vi "CIPT_softwarecontrol with trigger.vi"() -> ()   [LabVIEW 2022 SP3]
uses:
  Git/CIPT/CIPT/Labview Project/CIPT modes.ctl
  <vilib>/Analysis/baseanly.llb/Mean (DBL).vi
  <vilib>/Utility/file.llb/Read Delimited Spreadsheet (DBL).vi
  <vilib>/Utility/file.llb/Read Delimited Spreadsheet (I64).vi
  <vilib>/gmath/NumericalOptimization/Nonlinear Curve Fit LM.vi
  <vilib>/Utility/file.llb/Write Delimited Spreadsheet (string).vi
  <vilib>/Utility/file.llb/Write Delimited Spreadsheet (I64).vi
  <vilib>/Utility/file.llb/Write Delimited Spreadsheet (DBL).vi
  C:/CIPT/Labview Project/Camera Driver/Labview Driver/OtherDrivers/LabVIEW/ueye.NET/uEyeDotNet.dll
  CIPT/Labview Project/Camera Driver/Labview Driver/OtherDrivers/LabVIEW/ueye.NET/uEyeDotNet.dll
  <vilib>/gmath/NI_Gmath.lvlib
  <instrlib>/Keithley DMM6500 DAQ6500 Series/Keithley DMM6500 DAQ6500 Series.lvlib
  <instrlib>/Keithley 24XX/Keithley 24XX.lvlib
  <instrlib>/Keithley 2182/Keithley 2182.lvlib
  <vilib>/Analysis/NI_AALBase.lvlib
panel:
  out "Comms Errors":errorcluster[](array[cluster])
  in  "Save Filr":bool
  out "error file out":errorcluster
  in  "output file path":path=path "C:/CIPT/Labview Project/csv files/test output.csv"
  in  "stop":bool
  in  "Tab Control":T1(tab)
  in  "Camera ID 3":enum16{"2", "1"}(ring)
  in  "Camera ID 1":enum16{"2", "1"}(ring)
  in  "down a2":bool
  in  "up a2":bool
  in  "down a1":bool
  in  "up a1":bool
  in  "down a3":bool
  in  "up a3":bool
  in  "down all":bool
  in  "up all":bool
  in  "steps /\n continuous \ntoggle":bool
  out "Image first camera":picture
  out "Serial Number 1":string
  in  "Init Camera":bool
  in  "Exit Camera":bool
  in  "Init Camera 2":bool
  in  "Exit Camera 2":bool
  out "Serial Number 2":string
  out "Image second camera":picture
  out "Error Camera 1":errorcluster caption="error"
  out "Error Camera 2":errorcluster caption="error"
  in  "COM 1":refnum<visa-resource-name>
  out "error":errorcluster
  in  "Probe Landing File":path=path "C:/CIPT/Labview Project/csv files/Probe Landing cipt.csv"
  in  "Landing Test on/off?":bool
  in  "load file":bool
  in  "Step size":i32=10
  out "Resistance":dbl[][](array[numeric])
  out "Measurment":sgl[](array[numeric])
  out "Loaded":bool
  out "Loaded":bool
  out "Error Probe Configuration File":errorcluster
  in  "Probe Configuration File":path=path "C:/CIPT/Labview Project/csv files/test probe config.csv"
  in  "Probe Settings File":path=path "C:/CIPT/Labview Project/csv files/deafult_probe_setrings.CSV"
  out "Error Probe Settings File":errorcluster
  out "Probe Spacings":dbl[][](array[numeric])
  in  "Load":bool
  in  "Multiplexer":refnum<visa-resource-name>
  out "all rows":i64[][](array[numeric])
  out "Results Description":string[](array[string])
  out "Results":dbl[][](array[numeric])
  out "Probe Set 2":i32
  in  "Compliance voltage (V)":dbl=42.0
  in  "Measure Instrument":refnum<visa-resource-name>
  in  "Radio Buttons":T2 caption="Select Instrumentation"
  in  "Source Instrument":refnum<visa-resource-name>
  in  "Run":bool
  in  "Current (µA)":dbl=10.0
  out "Measurement Log":string
  out "Probe Set":i32
  in  "Measurement Repeats":i32=10
  in  "Size Of Buffer":i32=3
  in  "Time For Buffer To Fill(ms)":u32=2000
  in  "Top Film R est.":dbl=0.25
  in  "Bottm Film R est.":dbl=0.25
  in  "RA est.":dbl=0.25
  out "Top Film R":dbl
  out "Bottom Film R":dbl
  out "RA":dbl
  out "error out (fitting model)":errorcluster
  in  "Fit Data":bool
  out "Measurements Map Out":map{string, dbl[]}(c390)
  # "Probe Landing cipt_probe check: checks probes individually \nProbe Landing cipt: checks for any connection"
  # "All"
  # "End"
  # "home"
  # "Delete"
  # "Insert"
  # "Page Down"
  # "Page up"
  # "F2"
  # "F1"
  # "Steps"
  # "Continuous"
  # "Probe Settings"
  # "Probe Configuration"
  # "I+"
  # "V+"
  # "V-"
  # "I-"
  # "Max Resolution of 2400 is 300 µV in 200 mV range"
  # "/"
  # "Sheet Resistance (RA)"
  # "Estimated Values"
  # "Fitted Values"
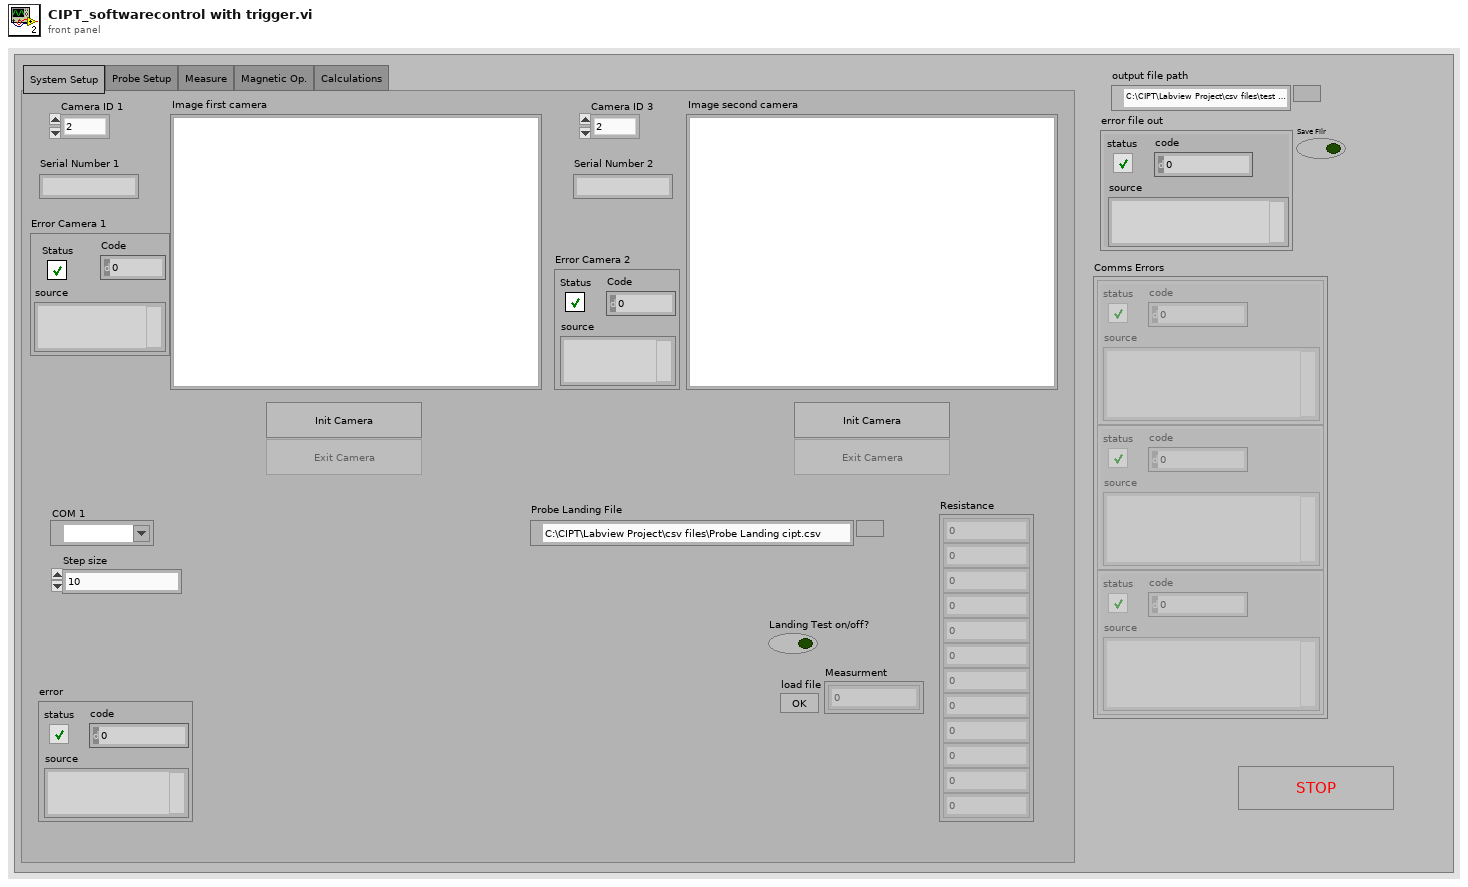
[diagram p1: front panel]
types:
  T1 = enum32{"System Setup", "Probe Setup", "Measure", "Magnetic Op.", "Calculations"}
  T2 = typedef "CIPT modes.ctl" = enum32{"DAQ6510", "2400 Only", "2400 and  2182", "SR830", "SR830 and 6221"}
  T3 = enum32{"System Setup", "Probe Setup", "Measure", "Magnetic Operations", "Calculations + Analyis"}
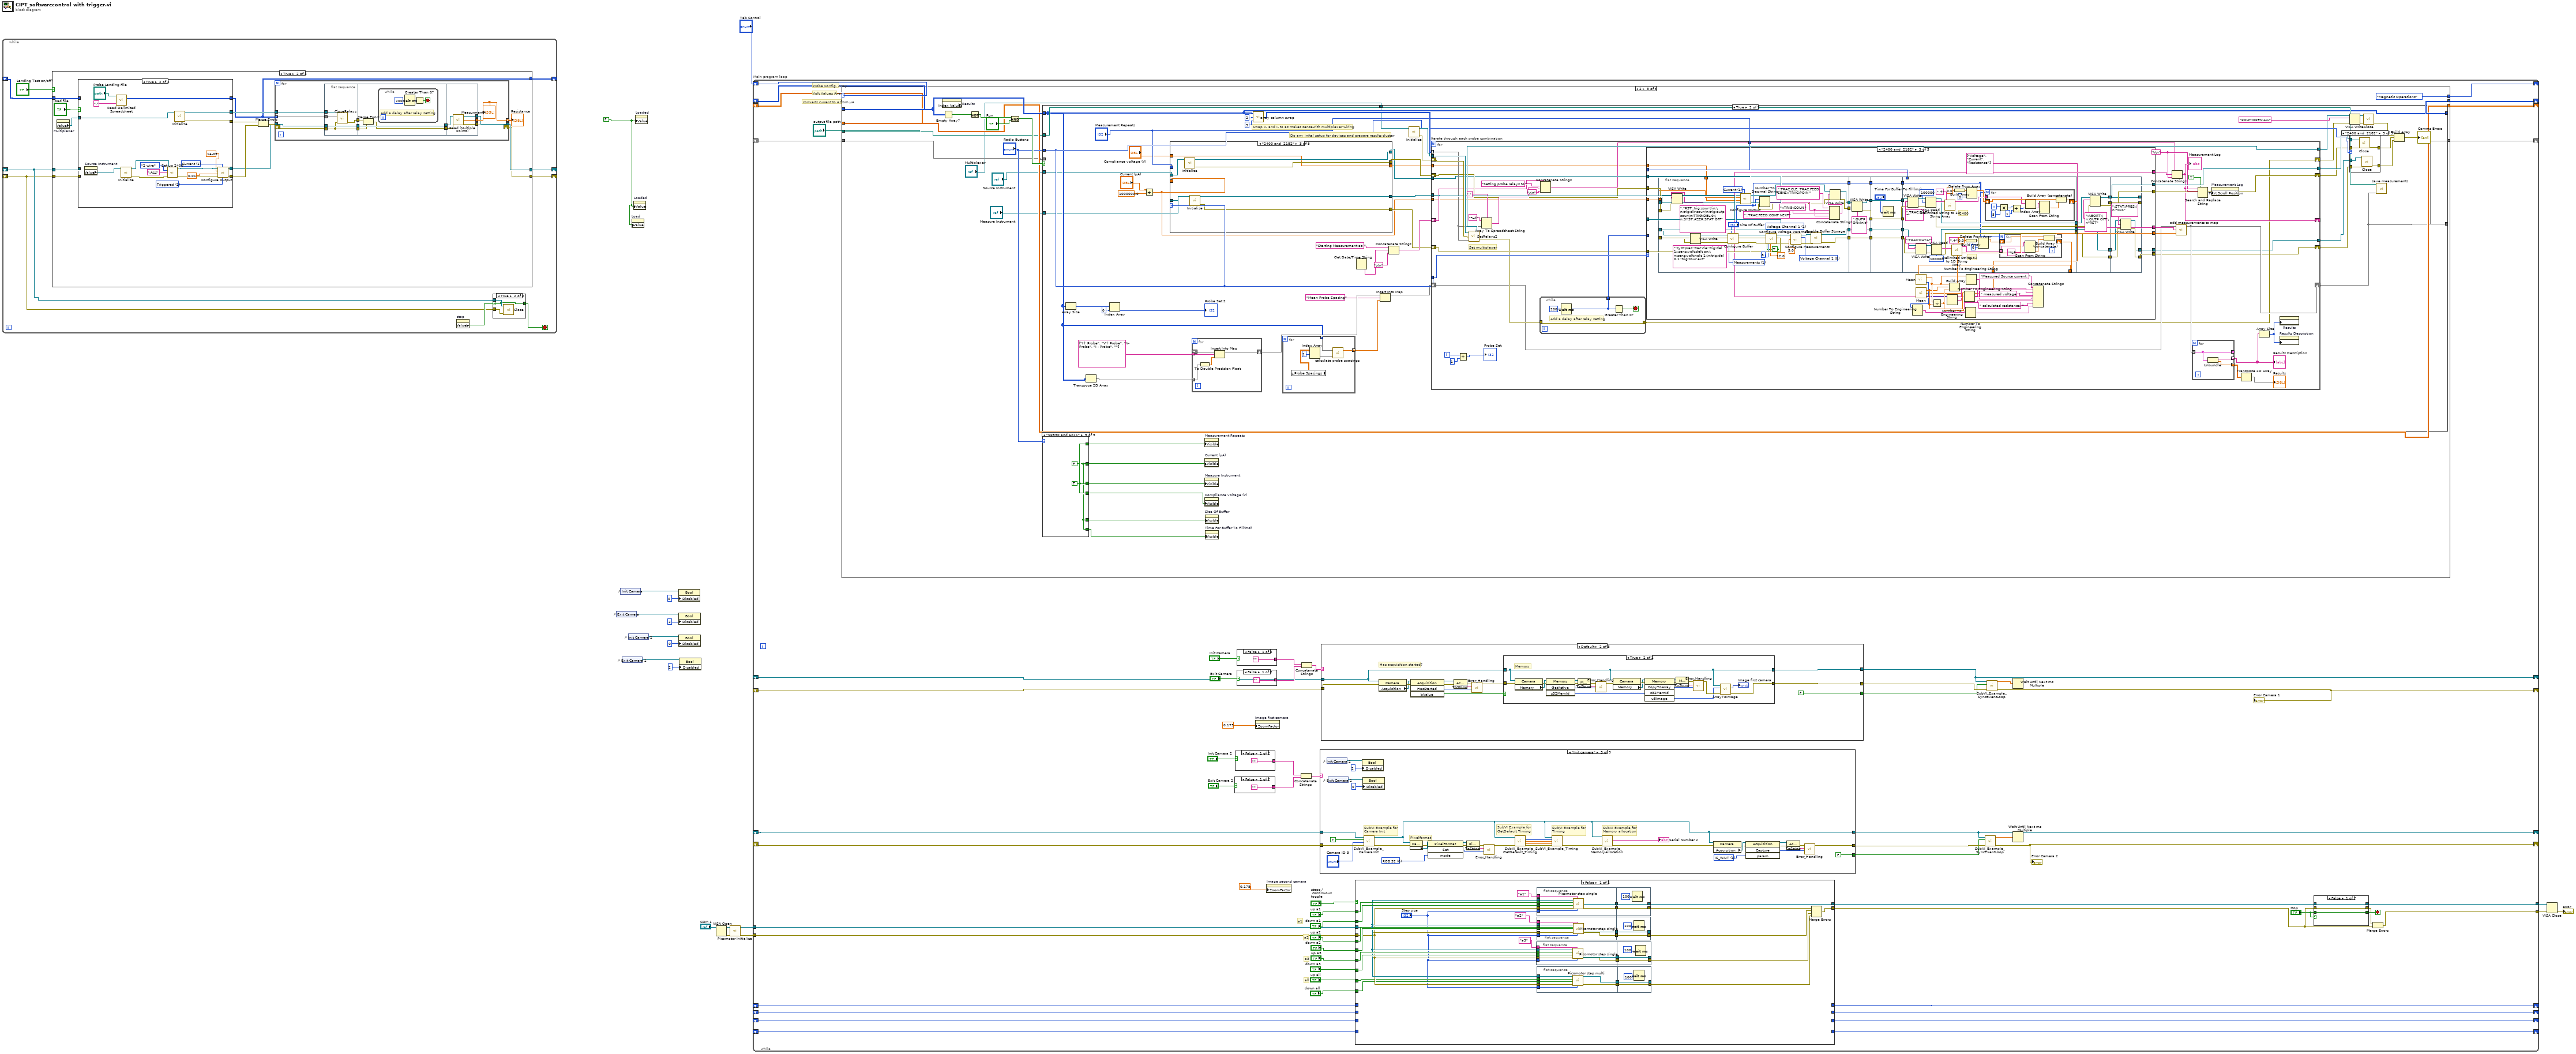
[diagram p0: block diagram]
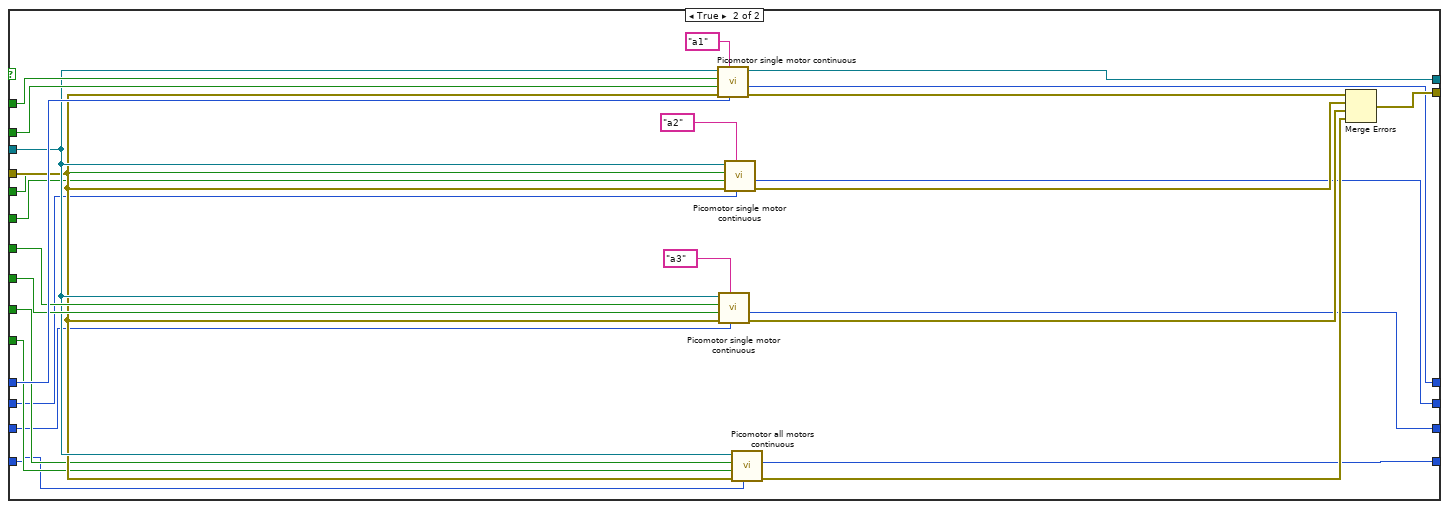
[diagram p5: hidden frame]
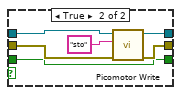
[diagram p6: hidden frame]
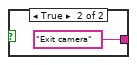
[diagram p7: hidden frame]
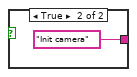
[diagram p8: hidden frame]
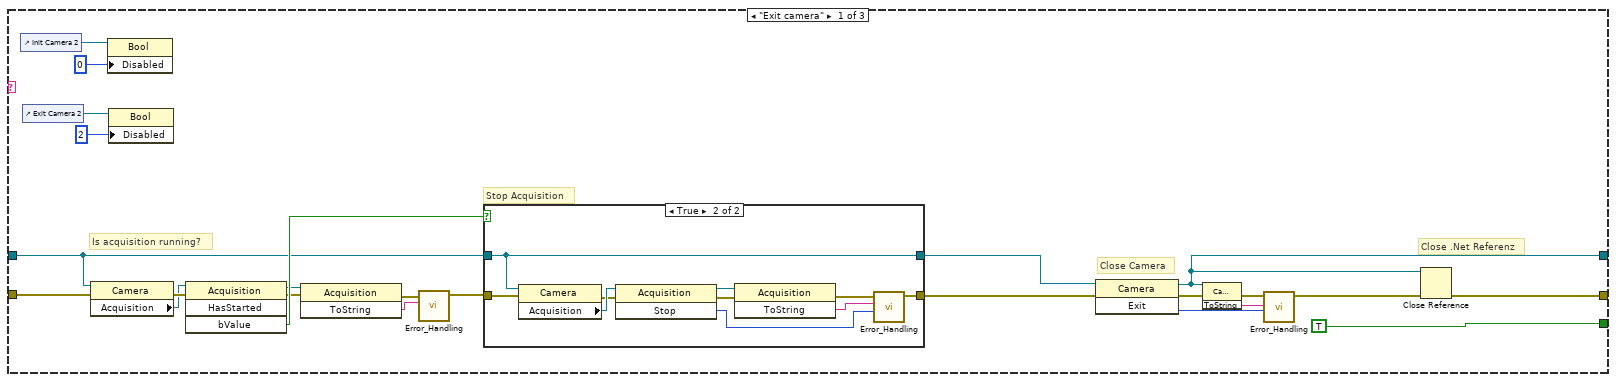
[diagram p9: hidden frame]
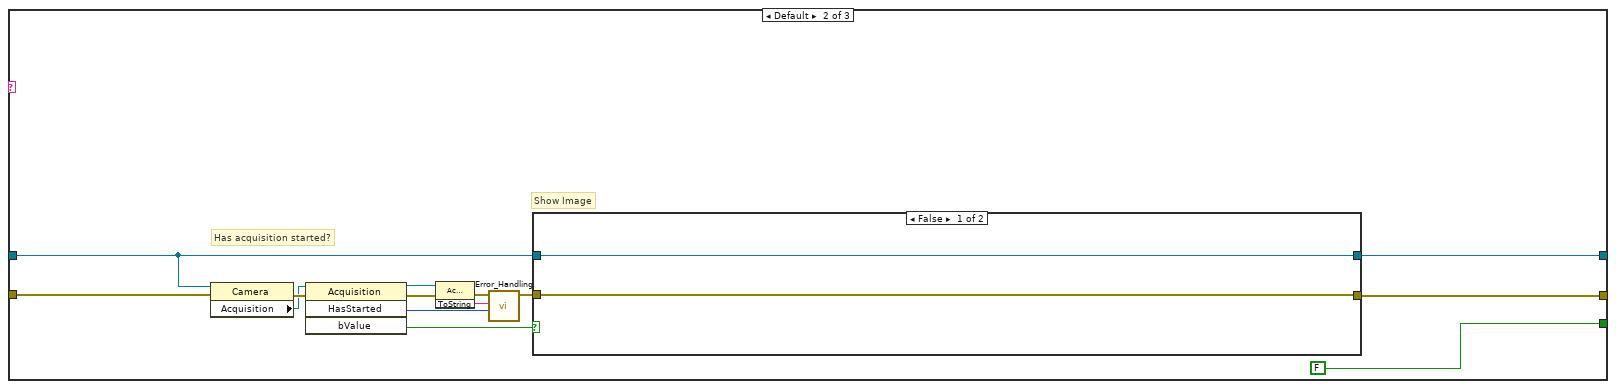
[diagram p11: hidden frame]
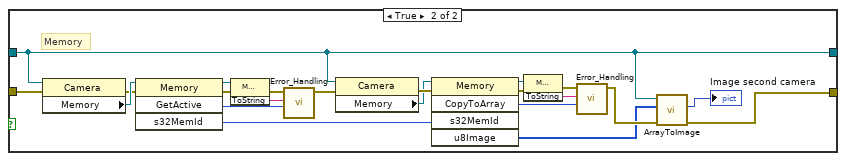
[diagram p12: hidden frame]
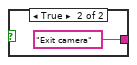
[diagram p13: hidden frame]
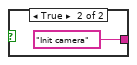
[diagram p14: hidden frame]
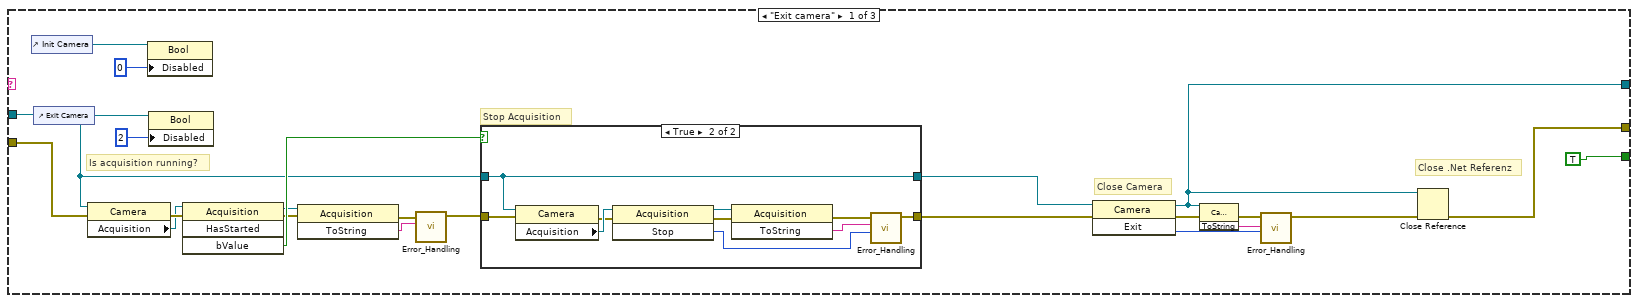
[diagram p15: hidden frame]
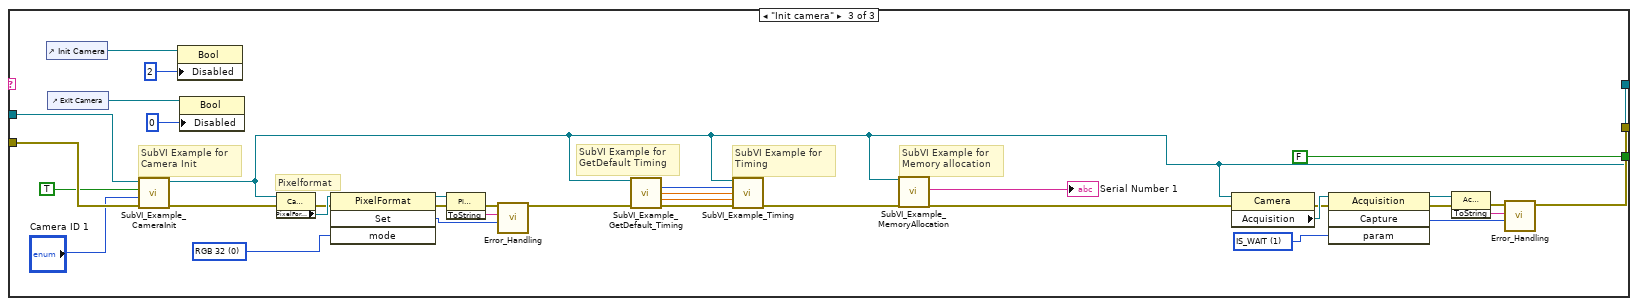
[diagram p18: hidden frame]
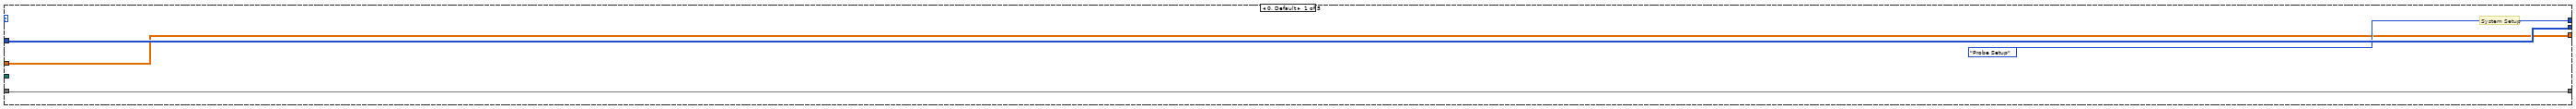
[diagram p19: hidden frame]
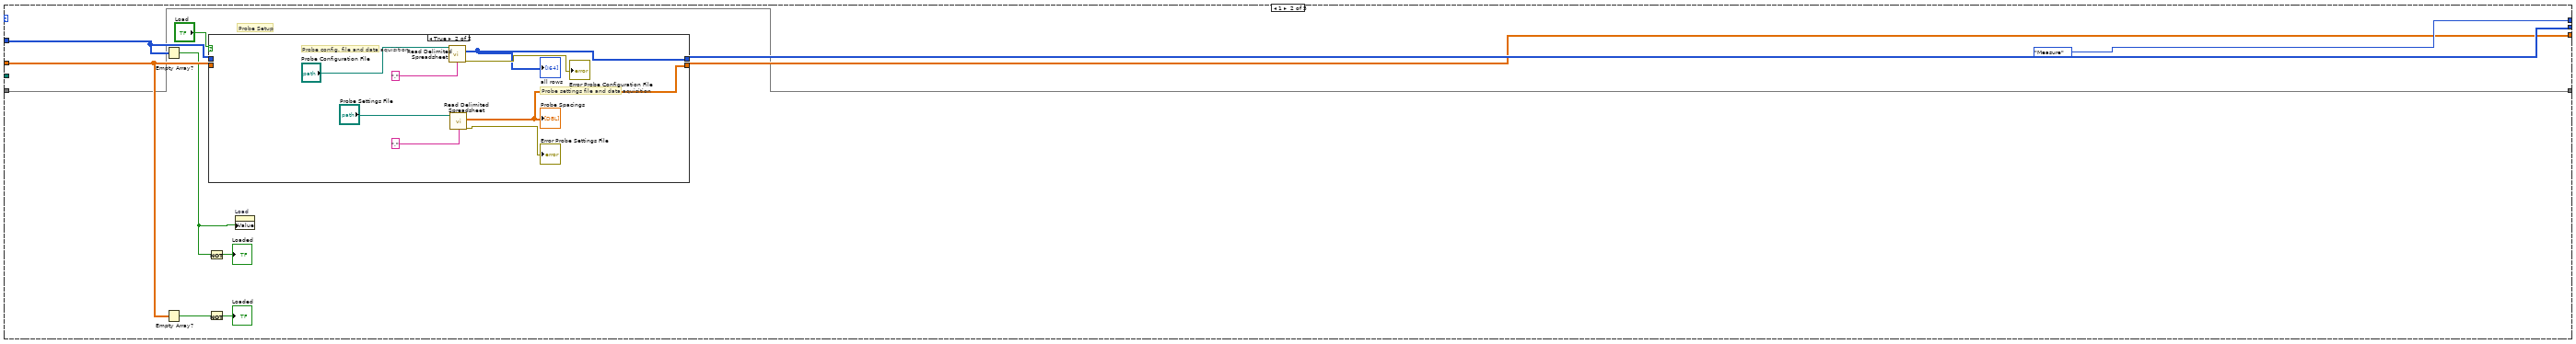
[diagram p20: hidden frame]
diagram:
  w9 = FALSE
  n1 = while {
    shift-right: [w26] -> _
    shift-left: _ -> [w23]
    shift-right: [w25] -> _
    shift-left: _ -> [w22]
    shift-right: [w20] -> _
    shift-left: _ -> [w19]
    stop <- w21 stop-if-true
    n2 = case shown="True" "Landing Test on/off?" {
      tunnel: w23 -> [w34 w43]
      tunnel: w22 -> [w33 w42]
      tunnel: [w34 w41] -> w26
      tunnel: [w33 w40] -> w25
      tunnel: w19 -> [w32 w36]
      tunnel: [w32 w35] -> w20
      frame False {
      }
      frame True {
        n3 = property on="Multiplexer" class="VISAName"() -> ("Value"=w39:refnum<visa-resource-name>)  [unwired: 2 in, 2 out]
        n4 = case shown="True" "load file" {
          tunnel: [_ w84] -> w48
          tunnel: [w80 w87] -> w45
          tunnel: [w81 w86] -> w44
          tunnel: w43 -> [w81 _]
          tunnel: w42 -> [w80 _]
          tunnel: [w79 w85] -> w38
          tunnel: w39 -> [w79 w83]
          tunnel: [w78 w82] -> w35
          tunnel: w36 -> [w78 _]
          frame False {
          }
          frame True {
            w93 = u16 1 items=["Immediate", "Triggered"] ("Output Type  (0: Immediate)")
            w92 = u16 1 items=["Voltage", "Current"] ("Source Mode  (0: Voltage)")
            n5 = property on="Source Instrument" class="VISAName"() -> ("Value"=w98:refnum<visa-resource-name>)  [unwired: 2 in, 2 out]
            n6 = call-poly <vilib>:"Read Delimited Spreadsheet.vi"("file path (dialog if empty)"="Probe Landing File", "delimiter (\\t)"="," ("delimiter (\\t)")) -> ("all rows"=w82:i64[][])  [unwired: 8 in, 5 out]
            n7 = call <instrlib>:"Initialize.vi"("VISA resource name"=w98) -> ("error out"=w95:errorcluster, "VISA resource name out"=w94:refnum<visa-resource-name>)  [unwired: 9 in]
            n8 = call "Set up 2400.vi"("VISA resource name"=w94, "Sense mode"=enum16{"2 wire", "4 wire"}."2 wire", "Measurement Function"=":ALL", "error in (no error)"=w95) -> ("VISA resource name out"=w96:refnum<visa-resource-name>, "error out"=w97:errorcluster)  [unwired: 10 in]
            n9 = call <instrlib>:"Initialize.vi"("VISA resource name"=w83) -> ("error out"=w84:errorcluster, "VISA resource name out"=w85:refnum<visa-resource-name>)  [unwired: 9 in]
            n10 = call <instrlib>:"Configure Output.vi"("Output Type  (0: Immediate)"=w93, "Source Mode  (0: Voltage)"=w92, "error in (no error)"=w97, "Compliance  Level (0.1)"=0.01, "Output Level (0)"=1e-05, "VISA resource name"=w96) -> ("error out"=w87:errorcluster, "VISA resource name out"=w86:refnum<visa-resource-name>)  [unwired: 4 in]
          }
        }
        n11 = Merge Errors(w48, w45) -> (w47:errorcluster)
        n12 = for {
          tunnel: [w54] -> w37 mode=indexing
          tunnel: w38 -> [w50]
          shift-right: [w51] -> w40
          shift-left: w47 -> [w55]
          tunnel: w35 -> [w49] mode=indexing
          tunnel: w44 -> [w53]
          tunnel: [w52] -> w41
          n13 = flat-sequence {
            tunnel: w53 -> [w65]
            tunnel: w55 -> [w61]
            tunnel: [w61] -> w60
            tunnel: [w65] -> w59
            tunnel: w50 -> [w64]
            tunnel: [w63] -> w58
            tunnel: w49 -> [w62]
            tunnel: [w67] -> w57
            tunnel: [w69] -> w56
            tunnel: w60 -> [w68]
            tunnel: w59 -> [w69]
            tunnel: w58 -> [w66]
            tunnel: [w75] -> w54
            tunnel: [w74] -> w52
            tunnel: [w73] -> w51
            tunnel: w57 -> [w77]
            tunnel: w56 -> [w76]
            frame #0 {
              n14 = call "CloseRelays.vi"("error in (no error)"=w61, "Array"=w62, "VISA Refnum in"=w64) -> ("error out"=w63:errorcluster)  [unwired: 6 in, 2 out]
            }
            frame #1 {
              n15 = Merge Errors(w66, w68) -> (w67:errorcluster)
              n16 = while {
                stop <- w71 stop-if-true
                # "Add a delay after relay setting"
                n17 = Wait (ms)(milliseconds to wait=u32 200) -> (millisecond timer value=w70:u32)
                n18 = Greater Than 0?(x=w70) -> (x > 0?=w71:bool)
              }
            }
            frame #2 {
              n19 = call <instrlib>:"Read (Multiple Points).vi"("VISA resource name"=w76, "error in (no error)"=w77) -> ("VISA resource name out"=w74:refnum<visa-resource-name>, "Resistance"=w75:sgl[], "error out"=w73:errorcluster)  [unwired: 7 in, 4 out]
            }
          }
          "Measurment" <- w54
        }
        "Resistance" <- w37
      }
    }
    n20 = property on="stop" class="Bool (strict)"() -> ("Value"=w24:bool)  [unwired: 2 in, 2 out]
    n21 = case shown="True" w24 {
      selector: w24 -> [w28 w29]
      tunnel: w23 -> [_ w31]
      tunnel: w22 -> [_ w30]
      tunnel: [w28 w29] -> w21
      frame False {
      }
      frame True {
        n22 = call <instrlib>:"Close.vi"("error in (no error)"=w30, "VISA resource name"=w31) -> ()  [unwired: 9 in, 1 out]
      }
    }
  }
  n23 = control-ref of="Exit Camera"() -> (w12:refnum<vi>)
  n24 = control-ref of="Init Camera"() -> (w13:refnum<vi>)
  n25 = control-ref of="Exit Camera 2"() -> (w17:refnum<vi>)
  n26 = control-ref of="Init Camera 2"() -> (w16:refnum<vi>)
  n27 = property on="Load" class="Bool (strict)"("Value"=w9) -> ()  [unwired: 2 in, 2 out]
  n28 = property on="Loaded" class="Bool (strict)"("Value"=w9) -> ()  [unwired: 2 in, 2 out]
  n29 = property on="Loaded" class="Bool (strict)"("Value"=w9) -> ()  [unwired: 2 in, 2 out]
  n30 = property class="Bool"(reference=w13, "Disabled"=u8 0 ("Deaktiviert")) -> ()  [unwired: 1 in, 2 out]
  n31 = property class="Bool"(reference=w12, "Disabled"=u8 2 ("Deaktiviert")) -> ()  [unwired: 1 in, 2 out]
  n32 = property class="Bool"(reference=w16, "Disabled"=u8 0 ("Deaktiviert")) -> ()  [unwired: 1 in, 2 out]
  n33 = property class="Bool"(reference=w17, "Disabled"=u8 2 ("Deaktiviert")) -> ()  [unwired: 1 in, 2 out]
  n34 = VISA Open(VISA resource name="COM 1") -> (VISA resource name=w7:refnum<visa-resource-name>, error out=w6:errorcluster)  [unwired: 4 in]
  n35 = call "Picomotor Initialize.vi"("error in (no error)"=w6, "VISA Refnum in"=w7) -> ("error out"=w4:errorcluster, "VISA Refnum out"=w5:refnum<visa-resource-name>)  [unwired: 8 in]
  n36 = while "Main program loop" {
    shift-right: [w159] -> _
    shift-left: _ -> [w160]
    shift-right: [w158] -> _
    shift-left: "Tab Control" -> [w161]
    shift-right: [w157] -> _
    shift-left: _ -> [w156]
    shift-right: [w154] -> _
    shift-left: _ -> [w153]
    shift-right: [w142] -> _
    shift-left: _ -> [w140]
    shift-right: [w143] -> _
    shift-left: _ -> [w141]
    shift-right: [w130] -> _
    shift-left: _ -> [w128]
    shift-right: [w129] -> _
    shift-left: _ -> [w127]
    tunnel: w5 -> [w114]
    tunnel: w4 -> [w113]
    tunnel: [w126] -> w2
    shift-right: [w111] -> _
    shift-left: _ -> [w107]
    shift-right: [w110] -> _
    shift-left: _ -> [w106]
    shift-right: [w109] -> _
    shift-left: _ -> [w105]
    shift-right: [w108] -> _
    shift-left: _ -> [w104]
    tunnel: [w101] -> w1
    stop <- w125 stop-if-true
    # "a2"
    # "a3"
    # "all"
    # "a1"
    # "converts current to A from µA"
    # "Volt Values Array"
    # "Probe Config. Array"
    n37 = case shown="2" w161 {
      tunnel: w160 -> [w500 w507 w538 w895 w902]
      tunnel: [w500 w511 w537 w895 w902] -> w159
      tunnel: [T3."Probe Setup" ("Tab Control") T3."Measure" ("Tab Control") T3."Magnetic Operations" ("Tab Control") T3."Calculations + Analyis" ("Tab Control") T3."System Setup" ("Tab Control")] -> w158
      tunnel: [w498 w506 w532 w894 w901] -> w157
      tunnel: w156 -> [w498 w505 w532 w894 w901]
      tunnel: "output file path" -> [_ _ w530 _ w900]
      tunnel: [w497 w502 w529 w893 w899] -> w154
      tunnel: w153 -> [w497 w502 w528 w893 w899]
      frame 0, Default {
        # "System Setup"
      }
      frame 1 {
        # "Probe Setup"
        n38 = Empty Array?(array=w507) -> (empty?=w501:bool)
        n39 = Empty Array?(array=w505) -> (empty?=w504:bool)
        n40 = Not(x=w501) -> (.not. x?=→"Loaded":bool)
        n41 = Not(x=w504) -> (.not. x?=→"Loaded":bool)
        n42 = case shown="True" "Load" {
          tunnel: [w513 w514] -> w511
          tunnel: w507 -> [w513 _]
          tunnel: [w512 w515] -> w506
          tunnel: w505 -> [w512 _]
          frame False {
          }
          frame True {
            # "Probe config. file and data aquisition"
            # "Probe settings file and data aquisition"
            n43 = call-poly <vilib>:"Read Delimited Spreadsheet.vi"("file path (dialog if empty)"="Probe Configuration File", "delimiter (\\t)"="," ("delimiter (\\t)")) -> ("all rows"=w514:i64[][], "error out"=→"Error Probe Configuration File":errorcluster)  [unwired: 8 in, 4 out]
            "all rows" <- w514
            n44 = call-poly <vilib>:"Read Delimited Spreadsheet.vi"("file path (dialog if empty)"="Probe Settings File", "delimiter (\\t)"="," ("delimiter (\\t)")) -> ("all rows"=w515:dbl[][], "error out"=→"Error Probe Settings File":errorcluster)  [unwired: 8 in, 4 out]
            "Probe Spacings" <- w515
          }
        }
        n45 = property on="Load" class="Bool (strict)"("Value"=w501) -> ()  [unwired: 2 in, 2 out]
      }
      frame 2 {
        n46 = property on="Results" class="Arr (strict)" props=["Index Values"]() -> ()  [unwired: 2 in, 3 out]
        n47 = Empty Array?(array=w538) -> (empty?=w540:bool)
        n48 = Not(x=w540) -> (.not. x?=w539:bool)
        n49 = Compound Arithmetic op=AND(w539, "Run") -> (w542:bool)
        n50 = case shown="True" w542 {
          tunnel: w538 -> [w553 w572]
          tunnel: [w553 w572] -> w537
          tunnel: "Radio Buttons" -> [_ w598]
          tunnel: w530 -> [_ w586]
          tunnel: [w552 w568] -> w529
          tunnel: w528 -> [w552 _]
          tunnel: "Measure Instrument" -> [_ w560]
          tunnel: "Source Instrument" -> [_ w559]
          tunnel: "Multiplexer" -> [_ w558]
          frame False {
          }
          frame True {
            # "Swap V- and I- to as makes sensewith multiplexer wiring"
            # "Do any inital setup for devices and prepare results cluster"
            n51 = Array Size(array=w572) -> (size(s)=w592:i32[])
            n52 = Transpose 2D Array(2D array=w572) -> (transposed array=w571:i64[][])
            n53 = Index Array "Index Array"(array=w592, index=0) -> (element=→"Probe Set 2":i32)
            n54 = Divide(x="Current (µA)", y=1000000.0) -> (x/y=w554:dbl)
            n55 = case shown="\"2400 and  2182\"" w598 {
              tunnel: w559 -> [_ w636 w642 _ _]
              tunnel: [_ w624 w641 _ _] -> w599
              tunnel: w560 -> [_ _ w643 _ _]
              tunnel: [_ w624 w639 _ _] -> w562
              tunnel: [_ w630 w638 _ _] -> w593
              tunnel: w554 -> [_ w627 _ _ _]
              tunnel: "Compliance voltage (V)" -> [_ w625 w637 _ _]
              tunnel: "Measurement Repeats" -> [_ _ _ _ _]
              tunnel: [_ _ w640 _ _] -> w557
              tunnel: [_ _ w637 _ _] -> w555
              frame "DAQ6510", Default {
              }
              frame "2400 Only" {
                w628 = u16 1 items=["Immediate", "Triggered"] ("Output Type  (0: Immediate)")
                w629 = u16 1 items=["Voltage", "Current"] ("Source Mode  (0: Voltage)")
                n56 = call <instrlib>:"Initialize.vi"("VISA resource name"=w636) -> ("error out"=w634:errorcluster, "VISA resource name out"=w635:refnum<visa-resource-name>)  [unwired: 9 in]
                n57 = call "Set up 2400.vi"("VISA resource name"=w635, "Sense mode"=enum16{"2 wire", "4 wire"}."4 wire", "Measurement Function"=":ALL", "error in (no error)"=w634) -> ("VISA resource name out"=w632:refnum<visa-resource-name>, "error out"=w631:errorcluster)  [unwired: 10 in]
                n58 = call <instrlib>:"Configure Output.vi"("Output Type  (0: Immediate)"=w628, "Source Mode  (0: Voltage)"=w629, "error in (no error)"=w631, "Compliance  Level (0.1)"=w625, "Output Level (0)"=w627, "VISA resource name"=w632) -> ("error out"=w630:errorcluster, "VISA resource name out"=w624:refnum<visa-resource-name>)  [unwired: 4 in]
              }
              frame "2400 and  2182" {
                n59 = call <instrlib>:"Initialize.vi"("VISA resource name"=w642) -> ("error out"=w638:errorcluster, "VISA resource name out"=w639:refnum<visa-resource-name>)  [unwired: 9 in]
                n60 = call <instrlib>:"Initialize.vi"("VISA resource name"=w643) -> ("error out"=w640:errorcluster, "VISA resource name out"=w641:refnum<visa-resource-name>)  [unwired: 9 in]
              }
              frame "SR830" {
              }
              frame "SR830 and 6221" {
              }
            }
            n61 = for {
              tunnel: w571 -> [w610] mode=indexing
              tunnel: string[] ["I+ Probe", "V+ Probe", "V- Probe", "I - Probe", ""] -> [w611] mode=indexing
              shift-right: [w608] -> w576
              shift-left: _ -> [w607]
              n62 = To Double Precision Float(number=w610) -> (double precision float=w609:dbl[])
              n63 = Insert Into Map(map in=w607, key=w611, value=w609) -> (map out=w608:map{string, dbl[]})  [unwired: 2 out]
            }
            n64 = call "array column swap.vi"("Collumn 2 index"=3, "Collumn 1 index"=2, "Input array"=w572) -> ("output array"=w589:i32[][])
            n65 = for {
              tunnel: w572 -> [w603] mode=indexing
              tunnel: [w602] -> w575 mode=indexing
              n66 = local read "Probe Spacings"() -> (w606:dbl[][])
              n67 = Index Array(array=w606, index (row)=1) -> (element=w604:dbl[])  [unwired: 1 in]
              n68 = call "calculate probe spacings.vi"("Probe Spacings"=w604, "Probe list"=w603) -> ("Mean Spacing"=w602:dbl)  [unwired: 1 out]
            }
            n69 = Get Date/Time String() -> (time string=w595:string)  [unwired: 3 in, 1 out]
            n70 = Insert Into Map(map in=w576, key="Mean Probe Spacing", value=w575) -> (map out=w573:map{string, dbl[]})  [unwired: 2 out]
            n71 = Concatenate Strings("Starting Measurement at: ", w595, "\r\n") -> (w584:string)
            n72 = call <instrlib>:"Initialize.vi"("VISA resource name"=w558) -> ("error out"=w600:errorcluster, "VISA resource name out"=w601:refnum<visa-resource-name>)  [unwired: 9 in]
            n73 = for "Iterate through each probe combination" {
              tunnel: w601 -> [w685]
              tunnel: [w684] -> w582
              tunnel: w589 -> [w678] mode=indexing
              tunnel: w598 -> [w683]
              tunnel: w599 -> [w681]
              shift-right: [w667] -> _
              shift-left: w584 -> [w668]
              shift-right: [w679] -> w596
              shift-left: w593 -> [w672]
              shift-right: [w658] -> w568
              shift-left: w573 -> [w660]
              shift-right: [w651] -> w569
              shift-left: w557 -> [w652]
              tunnel: w562 -> [w671]
              tunnel: [w680] -> w597
              shift-right: [w654] -> w564
              shift-left: w600 -> [w682]
              tunnel: [w650] -> w570
              tunnel: "Measurement Repeats" -> [w649]
              tunnel: w555 -> [w645]
              tunnel: w554 -> [w644]
              i -> [w648]
              w665 = "\r\n"
              # "Set multiplexer"
              n74 = Add(x=w648, y=1) -> (x+y=→"Probe Set":i32)
              n75 = call "SetRelays2.vi"("all rows"=w678, "error in (no error)"=w682, "VISA Refnum in"=w685) -> ("error out"=w673:errorcluster, "VISA resource name out"=w684:refnum<visa-resource-name>)  [unwired: 1 in]
              n76 = Array To Spreadsheet String(delimiter (Tab)=",", array=w678, 3:"%d" ("format string")) -> (spreadsheet string=w674:string)
              n77 = while {
                tunnel: [w692] -> w654
                tunnel: w673 -> [w692]
                tunnel: [w689] -> w653
                stop <- w690 stop-if-true
                # "Add a delay after relay setting"
                n78 = Wait (ms)(milliseconds to wait=u32 200) -> (millisecond timer value=w689:u32)
                n79 = Greater Than 0?(x=w689) -> (x > 0?=w690:bool)
              }
              n80 = Concatenate Strings(w668, "Setting probe relays to:", w674, "\r\n") -> (w663:string)
              n81 = case shown="\"2400 and  2182\"" w683 {
                tunnel: w681 -> [w694 w698 w763 w885 w889]
                tunnel: w671 -> [w693 w719 w771 w886 w890]
                tunnel: w672 -> [w695 w718 w770 w887 w891]
                tunnel: [w693 w716 w731 w886 w890] -> w680
                tunnel: [w695 w715 w739 w887 w891] -> w679
                tunnel: [_ w708 w764 _ _] -> w669
                tunnel: w649 -> [_ w707 w769 _ _]
                tunnel: [_ w701 w768 _ _] -> w661
                tunnel: [_ string[] ["Voltage", "Current", "Resistance"] string[] ["Voltage", "Current", "Resistance"] _ _] -> w662
                tunnel: w653 -> [_ _ _ _ _]
                tunnel: w652 -> [w696 w699 w762 w888 w892]
                tunnel: [w696 w699 w735 w888 w892] -> w651
                tunnel: [w694 w698 w732 w885 w889] -> w650
                tunnel: w645 -> [_ _ w724 _ _]
                tunnel: w644 -> [_ _ w723 _ _]
                frame "DAQ6510", Default {
                }
                frame "2400 Only" {
                  w717 = u16 0 items=["Fixed", "Sweep", "List"] ("Output Mode (0: Fixed)")
                  n82 = call <instrlib>:"Read (Multiple Points).vi"("VISA resource name"=w719, "Sample Count (1)"=w707, "error in (no error)"=w718, "Output Mode (0: Fixed)"=w717) -> ("Voltage"=w697:sgl[], "VISA resource name out"=w716:refnum<visa-resource-name>, "Current"=w706:sgl[], "Resistance"=w705:sgl[], "error out"=w715:errorcluster)  [unwired: 5 in, 2 out]
                  n83 = call-poly <vilib>:"Mean.vi"("X"=w697) -> ("mean"=w704:dbl)  [unwired: 1 out]
                  n84 = call-poly <vilib>:"Mean.vi"("X"=w706) -> ("mean"=w703:dbl)  [unwired: 1 out]
                  n85 = call-poly <vilib>:"Mean.vi"("X"=w705) -> ("mean"=w702:dbl)  [unwired: 1 out]
                  n86 = Build Array(w704, w703, w702) -> (w701:dbl[])
                  n87 = Number To Engineering String(4:w704) -> (0:w709:string)  [unwired: 3 in]
                  n88 = Number To Engineering String(4:w703) -> (0:w713:string)  [unwired: 3 in]
                  n89 = Number To Engineering String(4:w702) -> (0:w710:string)  [unwired: 3 in]
                  n90 = Concatenate Strings("Measured I = ", w713, " V = " ("string"), w709, "R = " ("string"), w710) -> (w708:string)
                }
                frame "2400 and  2182" {
                  n91 = flat-sequence {
                    tunnel: w762 -> [w785]
                    tunnel: w763 -> [w786]
                    tunnel: w770 -> [w778]
                    tunnel: w771 -> [w779]
                    tunnel: [w783] -> w734
                    tunnel: [w782] -> w733
                    tunnel: [w781] -> w726
                    tunnel: [w780] -> w725
                    tunnel: w724 -> [w776]
                    tunnel: w723 -> [w775]
                    tunnel: ["Size Of Buffer"] -> w720
                    tunnel: [w816] -> w751
                    tunnel: [w815] -> w749
                    tunnel: [w813] -> w746
                    tunnel: [w812] -> w744
                    tunnel: w734 -> [w816]
                    tunnel: w733 -> [w815]
                    tunnel: w726 -> [w814]
                    tunnel: w725 -> [_]
                    tunnel: [w810] -> w721
                    tunnel: w720 -> [w810]
                    tunnel: w751 -> [w822]
                    tunnel: [w822] -> w750
                    tunnel: w749 -> [w821]
                    tunnel: [w821] -> w748
                    tunnel: [w820] -> w747
                    tunnel: w746 -> [w820]
                    tunnel: [w819] -> w745
                    tunnel: w744 -> [w819]
                    tunnel: [w818] -> w722
                    tunnel: w721 -> [w818]
                    tunnel: w769 -> [_]
                    tunnel: w750 -> [w832]
                    tunnel: w748 -> [w831]
                    tunnel: w747 -> [w834]
                    tunnel: w745 -> [w833]
                    tunnel: [w830] -> w743
                    tunnel: [w829] -> w742
                    tunnel: [w827] -> w741
                    tunnel: [w826] -> w740
                    tunnel: [w825] -> w737
                    tunnel: [w824] -> w736
                    tunnel: w722 -> [w823]
                    tunnel: w741 -> [w877]
                    tunnel: w740 -> [w876]
                    tunnel: w737 -> [w872]
                    tunnel: w736 -> [w873]
                    tunnel: [w874] -> w730
                    tunnel: [w873] -> w729
                    tunnel: [w872] -> w728
                    tunnel: [w871] -> w727
                    tunnel: [w883] -> w731
                    tunnel: [w878] -> w732
                    tunnel: [w879] -> w735
                    tunnel: [w884] -> w739
                    tunnel: w730 -> [w884]
                    tunnel: w729 -> [w880]
                    tunnel: w728 -> [w881]
                    tunnel: w727 -> [w883]
                    frame #0 {
                      w787 = 0 items=["Voltage Channel 1", "Voltage Channel 2", "Temperature Channel 1", "Temperature Channel 2"] ("Measurement (0: Voltage Channel 1)")
                      w777 = u16 1 items=["Voltage", "Current"] ("Source Mode  (0: Voltage)")
                      w800 = 1 items=["Voltage Channel 1"=1, "Voltage Channel 2"=2] ("Measurement (1: Voltage Channel 1)")
                      w801 = 1 items=["None", "Measurements", "Math Calculation"] ("Buffer Source (0: None)")
                      n92 = VISA Write(VISA resource name=w779, write buffer=":*RST;:trig:sour tlin;\n:trig:dir sour;\n:trig:outp sour;\n:TRIG:DEL 0;\n:SYST:AZER:STAT OFF", error in (no error)=w778) -> (VISA resource name out=w796:refnum<visa-resource-name>, error out=w791:errorcluster)  [unwired: 1 out]
                      n93 = VISA Write(VISA resource name=w786, write buffer=":syst:pres;:trac:cle;:trig:del 1;:sens:volt:delt on;\n:sens:volt:nplc 1;\n:trig:del 0.1;:trig:sour ext", error in (no error)=w785) -> (VISA resource name out=w798:refnum<visa-resource-name>, error out=w797:errorcluster)  [unwired: 1 out]
                      n94 = call <instrlib>:"Configure Buffer.vi"("error in (no error)"=w797, "Buffer Source (0: None)"=w801, "Buffer Size (2)"="Size Of Buffer", "VISA resource name"=w798) -> ("error out"=w802:errorcluster, "VISA resource name out"=w805:refnum<visa-resource-name>)  [unwired: 6 in]
                      n95 = call <instrlib>:"Configure Output.vi"("Source Mode  (0: Voltage)"=w777, "error in (no error)"=w791, "Compliance  Level (0.1)"=w776, "Output Level (0)"=w775, "VISA resource name"=w796) -> ("error out"=w790:errorcluster, "VISA resource name out"=w774:refnum<visa-resource-name>)  [unwired: 5 in]
                      n96 = Number To Decimal String(number="Size Of Buffer") -> (decimal integer string=w792:string)  [unwired: 1 in]
                      n97 = call <instrlib>:"Configure Voltage Parameters.vi"("VISA resource name"=w805, "Measurement (1: Voltage Channel 1)"=w800, "Voltage Resolution (8)"=8, "Range Value (12)"=12.0, "Autorange (T: Enable)"=TRUE, "error in (no error)"=w802) -> ("VISA resource name out"=w804:refnum<visa-resource-name>, "error out"=w803:errorcluster)  [unwired: 8 in]
                      n98 = call <instrlib>:"Configure Measurements.vi"("VISA resource name"=w804, "Measurement (0: Voltage Channel 1)"=w787, "Integration Rate (5)"=5.0, "error in (no error)"=w803) -> ("VISA resource name out"=w789:refnum<visa-resource-name>, "error out"=w788:errorcluster)  [unwired: 10 in]
                      n99 = call <instrlib>:"Enable Buffer Storage.vi"("error in (no error)"=w788, "VISA resource name"=w789) -> ("error out"=w782:errorcluster, "VISA resource name out"=w783:refnum<visa-resource-name>)  [unwired: 8 in]
                      n100 = Concatenate Strings(":TRAC:CLE;:TRAC:FEED SENS;:TRAC:POIN " ("write buffer"), w792, ";:TRIG:COUN " ("write buffer"), w792, ";:TRAC:FEED:CONT NEXT" ("write buffer")) -> (w773:string)
                      n101 = VISA Write(VISA resource name=w774, write buffer=w773, error in (no error)=w790) -> (VISA resource name out=w781:refnum<visa-resource-name>, error out=w780:errorcluster)  [unwired: 1 out]
                    }
                    frame #1 {
                      n102 = VISA Write(VISA resource name=w814, write buffer=":OUTP ON;:init") -> (VISA resource name out=w813:refnum<visa-resource-name>, error out=w812:errorcluster)  [unwired: 1 in, 1 out]
                    }
                    frame #2 {
                      n103 = Wait (ms)(milliseconds to wait="Time For Buffer To Fill(ms)") -> ()  [unwired: 1 out]
                    }
                    frame #3 {
                      # "2182"
                      # "2400"
                      n104 = VISA Write(VISA resource name=w834, write buffer=":TRAC:DATA?", error in (no error)=w833) -> (VISA resource name out=w844:refnum<visa-resource-name>, error out=w843:errorcluster)  [unwired: 1 out]
                      n105 = VISA Write(VISA resource name=w832, write buffer=":TRAC:DATA?", error in (no error)=w831) -> (VISA resource name out=w853:refnum<visa-resource-name>, error out=w852:errorcluster)  [unwired: 1 out]
                      n106 = VISA Read(VISA resource name=w844, byte count=u32 100000, error in (no error)=w843) -> (VISA resource name out=w827:refnum<visa-resource-name>, read buffer=w840:string, error out=w826:errorcluster)  [unwired: 1 out]
                      n107 = VISA Read(VISA resource name=w853, byte count=u32 100000, error in (no error)=w852) -> (VISA resource name out=w825:refnum<visa-resource-name>, read buffer=w850:string, error out=w824:errorcluster)  [unwired: 1 out]
                      n108 = call <vilib>:"Delimited String to 1D String Array.vi"("delimiter"=",+" ("delimiter (Tab)"), "delimited string"=w840) -> ("string array"=w836:string[])  [unwired: 9 in]
                      n109 = call <vilib>:"Delimited String to 1D String Array.vi"("delimiter"=",+" ("delimiter (Tab)"), "delimited string"=w850) -> ("string array"=w845:string[])  [unwired: 9 in]
                      n110 = Build Array(0.0 ("array")) -> (w838:dbl[])
                      n111 = Build Array(0.0 ("array")) -> (w848:dbl[])
                      n112 = Delete From Array(array=w838, index=0) -> (array with subset deleted=w828:dbl[])  [unwired: 1 in, 1 out]
                      n113 = Delete From Array(array=w848, index=0) -> (array with subset deleted=w846:dbl[])  [unwired: 1 in, 1 out]
                      n114 = for {
                        N: w823 -> [_]
                        shift-right: [w859] -> w829
                        shift-left: w828 -> [w858]
                        tunnel: w836 -> [w857]
                        i -> [w865]
                        n115 = Multiply(x=w865, y=5) -> (x*y=w864:i32)
                        n116 = Add(x=w864, y=1) -> (x+y=w861:i32)
                        n117 = Index Array(array=w857, index=w861) -> (element=w856:string)
                        n118 = Scan From String(input string=w856) -> (output 1=w860:dbl)  [unwired: 4 in, 3 out]
                        n119 = Build Array (concatenate)(w858, w860) -> (w859:dbl[])
                      }
                      n120 = for {
                        N: w823 -> [_]
                        shift-right: [w868] -> w830
                        shift-left: w846 -> [w867]
                        tunnel: w845 -> [w866] mode=indexing
                        n121 = Scan From String(format string="%f", input string=w866) -> (output 1=w869:dbl)  [unwired: 3 in, 3 out]
                        n122 = Build Array (concatenate)(w867, w869) -> (w868:dbl[])
                      }
                    }
                    frame #4 {
                      n123 = VISA Write(VISA resource name=w877, write buffer=":ABORT;\n:OUTP OFF;\n*RST" ("data"), error in (no error)=w876) -> (VISA resource name out=w871:refnum<visa-resource-name>, error out=w874:errorcluster)  [unwired: 1 out]
                    }
                    frame #5 {
                      n124 = VISA Write(VISA resource name=w881, write buffer=":STAT:PRES;\n:*CLS" ("data"), error in (no error)=w880) -> (VISA resource name out=w878:refnum<visa-resource-name>, error out=w879:errorcluster)  [unwired: 1 out]
                    }
                  }
                  n125 = call-poly <vilib>:"Mean.vi"("X"=w743) -> ("mean"=w767:dbl, "error"=w755:i32)
                  n126 = Number To Engineering String(4:w755) -> (0:w754:string)  [unwired: 3 in]
                  n127 = call-poly <vilib>:"Mean.vi"("X"=w742) -> ("mean"=w766:dbl, "error"=w759:i32)
                  n128 = Divide(x=w767, y=w766) -> (x/y=w765:dbl)
                  n129 = Number To Engineering String(4:w759) -> (0:w758:string)  [unwired: 3 in]
                  n130 = Build Array(w767, w766, w765) -> (w768:dbl[])
                  n131 = Number To Engineering String(4:w766) -> (0:w760:string)  [unwired: 3 in]
                  n132 = Number To Engineering String(4:w765) -> (0:w752:string)  [unwired: 3 in]
                  n133 = Number To Engineering String(4:w767) -> (0:w756:string)  [unwired: 3 in]
                  n134 = Concatenate Strings("Measured Source current: " ("string"), w760, w758, " measured voltage: " ("string"), w756, w754, " calculated resistance: " ("string"), w752) -> (w764:string)
                }
                frame "SR830" {
                }
                frame "SR830 and 6221" {
                }
              }
              n135 = Concatenate Strings(w663, w669, w665) -> (w667:string)
              "Measurement Log" <- w667
              n136 = call "add measurements to map.vi"("Measurement Values"=w661, "Measurement Names"=w662, "Measurements Map in"=w660) -> ("Measurements Map Out"=w658:map{string, dbl[]})  [unwired: 2 in]
              n137 = for {
                tunnel: [w688] -> _ mode=indexing
                tunnel: w658 -> [w688] mode=indexing
                tunnel: [w687] -> w657 mode=indexing
                tunnel: [w686] -> w656 mode=indexing
                n138 = Unbundle(w688) -> (w687:string, "Array"=w686:dbl[])
              }
              "Results Description" <- w657
              n139 = Search and Replace String(replace all?=TRUE, input string=w667, search string=w665) -> (number of replacements=w664:i32)  [unwired: 5 in, 3 out]
              n140 = property on="Measurement Log" class="Str"("Text.Scroll Position"=w664) -> ()  [unwired: 2 in, 2 out]
              n141 = Transpose 2D Array(2D array=w656) -> (transposed array=→"Results":dbl[][])
              n142 = Array Size(array=w657) -> (size(s)=w659:i32)
              n143 = property on="Results" class="Arr (strict)"("Number of Columns"=w659) -> ()  [unwired: 2 in, 2 out]
              n144 = property on="Results Description" class="Arr (strict)"("Number of Columns"=w659) -> ()  [unwired: 2 in, 2 out]
            }
            n145 = VISA Write(VISA resource name=w582, write buffer="ROUT:OPEN:ALL", error in (no error)=w564) -> (VISA resource name out=w581:refnum<visa-resource-name>, error out=w580:errorcluster)  [unwired: 1 out]
            n146 = case shown="\"2400 and  2182\"" w598 {
              tunnel: w597 -> [_ w617 w622 _ _]
              tunnel: w596 -> [w613 w616 w623 _ _]
              tunnel: [w613 w615 w618 _ _] -> w567
              tunnel: w570 -> [_ _ w621 _ _]
              tunnel: w569 -> [w612 w614 w620 _ _]
              tunnel: [w612 w614 w619 _ _] -> w566
              frame "DAQ6510", Default {
              }
              frame "2400 Only" {
                n147 = call <instrlib>:"Close.vi"("error in (no error)"=w616, "VISA resource name"=w617) -> ("error out"=w615:errorcluster)  [unwired: 9 in]
              }
              frame "2400 and  2182" {
                n148 = call <instrlib>:"Close.vi"("error in (no error)"=w623, "VISA resource name"=w622) -> ("error out"=w618:errorcluster)  [unwired: 9 in]
                n149 = call <instrlib>:"Close.vi"("error in (no error)"=w620, "VISA resource name"=w621) -> ("error out"=w619:errorcluster)  [unwired: 9 in]
              }
              frame "SR830" {
              }
              frame "SR830 and 6221" {
              }
            }
            n150 = call <instrlib>:"Close.vi"("error in (no error)"=w580, "VISA resource name"=w581) -> ("error out"=w563:errorcluster)  [unwired: 9 in]
            n151 = call "save measurements.vi"("Save path"=w586, "Measurements In"=w568) -> ()  [unwired: 12 in, 2 out]
            n152 = Build Array(w563, w567, w566) -> (→"Comms Errors":errorcluster[])
          }
        }
        n153 = case shown="\"SR830 and 6221\"" "Radio Buttons" {
          tunnel: [w543 w545 w547 w548 w551] -> w536
          tunnel: [w543 w546 w547 w548 w550] -> w535
          tunnel: [TRUE w546 w547 TRUE w551] -> w531
          tunnel: [w543 w546 w547 w548 w551] -> w524
          tunnel: [w543 w545 w547 w548 w550] -> w523
          tunnel: [w543 w545 w547 w548 w550] -> w522
          frame "DAQ6510", Default {
            w543 = FALSE
          }
          frame "2400 Only" {
            w546 = TRUE
            w545 = FALSE
          }
          frame "2400 and  2182" {
            w547 = TRUE
          }
          frame "SR830" {
            w548 = FALSE
          }
          frame "SR830 and 6221" {
            w550 = FALSE
            w551 = TRUE
          }
        }
        n154 = property on="Measurement Repeats" class="DigNum (strict)"("Visible"=w531) -> ()  [unwired: 2 in, 2 out]
        n155 = property on="Current (µA)" class="DigNum (strict)"("Visible"=w535) -> ()  [unwired: 2 in, 2 out]
        n156 = property on="Measure Instrument" class="VISAName"("Visible"=w536) -> ()  [unwired: 2 in, 2 out]
        n157 = property on="Compliance voltage (V)" class="DigNum (strict)"("Visible"=w524) -> ()  [unwired: 2 in, 2 out]
        n158 = property on="Size Of Buffer" class="DigNum (strict)"("Visible"=w523) -> ()  [unwired: 2 in, 2 out]
        n159 = property on="Time For Buffer To Fill(ms)" class="DigNum (strict)"("Visible"=w522) -> ()  [unwired: 2 in, 2 out]
      }
      frame 3 {
        # "Magnetic Op."
      }
      frame 4 {
        # "Calculations"
        # "Save File - saves collected data into a (csv) file and asks for a file path if not already given"
        n160 = Look In Map(map=w899, key="Resistance") -> (value=w897:dbl[])  [unwired: 1 in, 1 out]
        n161 = Build Array("Top Film R est.", "Bottm Film R est.", "RA est.") -> (w907:dbl[])
        n162 = case shown="True" "Fit Data" {
          tunnel: w902 -> [_ w927]
          tunnel: w907 -> [_ w925]
          tunnel: [dbl[] [0.0, 0.0, 0.0] w916] -> w904
          tunnel: w897 -> [_ w914]
          frame False {
          }
          frame True {
            # "Calculated R"
            # "Mean probe spacing"
            n163 = Index Array(array=w927, index (col)=4 ("disabled index (col)")) -> (element=w926:i64[])  [unwired: 1 in]
            n164 = vi-ref "modelFunction.vi"() -> (w924:refnum<vi>)
            n165 = call-poly <vilib>:"Nonlinear Curve Fit.vi"("Y"=w914, "f(x,a)"=w924, "X"=w926, "initial parameters"=w925) -> ("best fit parameters"=w916:dbl[], "error out"=→"error out (fitting model)":errorcluster)  [unwired: 6 in, 4 out]
            n166 = Index Array(array=w916, index=0) -> (element=→"Top Film R":dbl)
            n167 = Index Array(array=w916, index=1) -> (element=→"Bottom Film R":dbl)
            n168 = Index Array(array=w916, index=2) -> (element=→"RA":dbl)
          }
        }
        n169 = case shown="True" "Save Filr" {
          tunnel: w902 -> [_ w948]
          tunnel: string[] ["I+", "V+", "V-", "I-", "x (mean probe spacing)", "V", "I (µA)", "R (=V/I)"] -> [_ w944]
          tunnel: string[] ["R (t)", "R (b)", "RA"] -> [_ w936]
          tunnel: w904 -> [_ w929]
          tunnel: w900 -> [_ w928]
          frame False {
          }
          frame True {
            n170 = call-poly <vilib>:"Write Delimited Spreadsheet.vi"("file path (dialog if empty)"=w928, "1D data"=w944, "delimiter (\\t)"="," ("delimiter (\\t)")) -> ("new file path (Not A Path if cancelled)"=w946:path, "error out"=w945:errorcluster)  [unwired: 11 in]
            n171 = call-poly <vilib>:"Write Delimited Spreadsheet.vi"("file path (dialog if empty)"=w946, "format (%d)"="%.6f" ("format (%.3f)"), "2D data"=w948, "append to file? (new file:F)"=TRUE, "error in (no error)"=w945, "delimiter (\\t)"="," ("delimiter (\\t)")) -> ("new file path (Not A Path if cancelled)"=w938:path, "error out"=w937:errorcluster)  [unwired: 8 in]
            n172 = call-poly <vilib>:"Write Delimited Spreadsheet.vi"("file path (dialog if empty)"=w938, "format (%s)"="%.6f" ("format (%.3f)"), "1D data"=w936, "append to file? (new file:F)"=TRUE, "error in (no error)"=w937, "delimiter (\\t)"="," ("delimiter (\\t)")) -> ("new file path (Not A Path if cancelled)"=w931:path, "error out"=w930:errorcluster)  [unwired: 8 in]
            n173 = call-poly <vilib>:"Write Delimited Spreadsheet.vi"("file path (dialog if empty)"=w931, "format (%.3f)"="%.6f", "1D data"=w929, "append to file? (new file:F)"=TRUE, "error in (no error)"=w930, "delimiter (\\t)"="," ("delimiter (\\t)")) -> ("error out"=→"error file out":errorcluster)  [unwired: 8 in, 1 out]
          }
        }
        "Measurements Map Out" <- w899
      }
    }
    n174 = case shown="False" "Exit Camera 2" {
      tunnel: ["" "Exit camera"] -> w135
      frame False {
      }
      frame True {
      }
    }
    n175 = case shown="False" "Init Camera 2" {
      tunnel: ["" "Init camera"] -> w138
      frame False {
      }
      frame True {
      }
    }
    n176 = case shown="False" "Init Camera" {
      tunnel: ["" "Init camera"] -> w151
      frame False {
      }
      frame True {
      }
    }
    n177 = case shown="False" "Exit Camera" {
      tunnel: ["" "Exit camera"] -> w148
      frame False {
      }
      frame True {
      }
    }
    n178 = property on="Image first camera" class="Pict"("ZoomFactor"=0.175) -> ()  [unwired: 2 in, 2 out]
    n179 = property on="Image second camera" class="Pict"("ZoomFactor"=0.175) -> ()  [unwired: 2 in, 2 out]
    n180 = Concatenate Strings(w138, w135) -> (w137:string)
    n181 = Concatenate Strings(w151, w148) -> (w150:string)
    n182 = case shown="\"Init camera\"" w137 {
      tunnel: w128 -> [w279 w310 w375]
      tunnel: w127 -> [w280 w309 w374]
      tunnel: [w289 w312 w353] -> w130
      tunnel: [w290 w311 w354] -> w134
      tunnel: [TRUE FALSE FALSE] -> w132
      frame "Exit camera" {
        # "Close .Net Referenz"
        # "Is acquisition running?"
        # "Stop Acquisition"
        # "Close Camera"
        n183 = control-ref of="Init Camera 2"() -> (w274:refnum<vi>)
        n184 = control-ref of="Exit Camera 2"() -> (w273:refnum<vi>)
        n185 = property class="Camera"(reference=w279, error in=w280) -> (error out=w288:errorcluster, "Acquisition"=w287:refnum<k24>)  [unwired: 1 out]
        n186 = property class="Bool"(reference=w274, "Disabled"=u8 0 ("Deaktiviert")) -> ()  [unwired: 1 in, 2 out]
        n187 = property class="Bool"(reference=w273, "Disabled"=u8 2 ("Deaktiviert")) -> ()  [unwired: 1 in, 2 out]
        n188 = invoke class="Acquisition" method="HasStarted"(reference=w287, error in=w288) -> (reference out=w281:refnum<k24>, error out=w284:errorcluster, "bValue"=w286:bool)  [unwired: 2 in, 1 out]
        n189 = invoke class="Acquisition" method="ToString"(reference=w281, error in=w284) -> (error out=w283:errorcluster, "ToString"=w282:string)  [unwired: 1 in, 1 out]
        n190 = call <instrlib>:"Error_Handling.vi"("Error String"=w282, "Error In"=w283) -> ("Error Out"=w285:errorcluster)  [unwired: 9 in]
        n191 = case shown="True" w286 {
          tunnel: [w298 w307] -> w277
          tunnel: w285 -> [w298 w308]
          tunnel: w279 -> [w297 w299]
          tunnel: [w297 w299] -> w278
          frame False {
          }
          frame True {
            n192 = property class="Camera"(reference=w299, error in=w308) -> (error out=w303:errorcluster, "Acquisition"=w304:refnum<k24>)  [unwired: 1 out]
            n193 = invoke class="Acquisition" method="Stop"(reference=w304, error in=w303) -> (reference out=w301:refnum<k24>, error out=w302:errorcluster, "Stop"=w300:i32)  [unwired: 1 in]
            n194 = invoke class="Acquisition" method="ToString"(reference=w301, error in=w302) -> (error out=w306:errorcluster, "ToString"=w305:string)  [unwired: 1 in, 1 out]
            n195 = call <instrlib>:"Error_Handling.vi"("Error Code"=w300, "Error String"=w305, "Error In"=w306) -> ("Error Out"=w307:errorcluster)  [unwired: 8 in]
          }
        }
        n196 = invoke class="Camera" method="Exit"(reference=w278, error in=w277) -> (reference out=w289:refnum<k24>, error out=w293:errorcluster, "Exit"=w292:i32)  [unwired: 1 in]
        n197 = invoke class="Camera" method="ToString"(reference=w289, error in=w293) -> (error out=w294:errorcluster, "ToString"=w295:string)  [unwired: 1 in, 1 out]
        n198 = call <instrlib>:"Error_Handling.vi"("Error Code"=w292, "Error String"=w295, "Error In"=w294) -> ("Error Out"=w291:errorcluster)  [unwired: 8 in]
        n199 = Close Reference ("Close Referenz")(reference=w289, error in (no error)=w291) -> (error out=w290:errorcluster)
      }
      frame Default {
        # "Has acquisition started?"
        # "Show Image"
        n200 = property class="Camera"(reference=w310, error in=w309) -> (error out=w321:errorcluster, "Acquisition"=w320:refnum<k24>)  [unwired: 1 out]
        n201 = invoke class="Acquisition" method="HasStarted"(reference=w320, error in=w321) -> (reference out=w316:refnum<k24>, error out=w315:errorcluster, "HasStarted"=w314:i32, "bValue"=w319:bool)  [unwired: 2 in]
        n202 = invoke class="Acquisition" method="ToString"(reference=w316, error in=w315) -> (error out=w318:errorcluster, "ToString"=w317:string)  [unwired: 1 in, 1 out]
        n203 = call <instrlib>:"Error_Handling.vi"("Error Code"=w314, "Error String"=w317, "Error In"=w318) -> ("Error Out"=w313:errorcluster)  [unwired: 8 in]
        n204 = case shown="False" w319 {
          tunnel: [w324 w330] -> w311
          tunnel: w313 -> [w324 w329]
          tunnel: w310 -> [w323 w325]
          tunnel: [w323 w325] -> w312
          frame False {
          }
          frame True {
            # "Memory"
            n205 = property class="Camera"(reference=w325, error in=w329) -> (error out=w332:errorcluster, "Memory"=w333:refnum<k24>)  [unwired: 1 out]
            n206 = invoke class="Memory" method="GetActive"(reference=w333, error in=w332) -> (reference out=w339:refnum<k24>, error out=w338:errorcluster, "GetActive"=w340:i32, "s32MemId"=w331:i32)  [unwired: 2 in]
            n207 = invoke class="Memory" method="ToString"(reference=w339, error in=w338) -> (error out=w336:errorcluster, "ToString"=w337:string)  [unwired: 1 in, 1 out]
            n208 = call <instrlib>:"Error_Handling.vi"("Error Code"=w340, "Error String"=w337, "Error In"=w336) -> ("Error Out"=w341:errorcluster)  [unwired: 8 in]
            n209 = property class="Camera"(reference=w325, error in=w341) -> (error out=w335:errorcluster, "Memory"=w334:refnum<k24>)  [unwired: 1 out]
            n210 = invoke class="Memory" method="CopyToArray"(reference=w334, error in=w335, "s32MemId"=w331) -> (reference out=w344:refnum<k24>, error out=w345:errorcluster, "CopyToArray"=w346:i32, "u8Image"=w326:u8[])  [unwired: 2 in, 1 out]
            n211 = invoke class="Memory" method="ToString"(reference=w344, error in=w345) -> (error out=w342:errorcluster, "ToString"=w343:string)  [unwired: 1 in, 1 out]
            n212 = call <instrlib>:"Error_Handling.vi"("Error Code"=w346, "Error String"=w343, "Error In"=w342) -> ("Error Out"=w327:errorcluster)  [unwired: 8 in]
            n213 = call <instrlib>:"ArrayToImage.vi"("Error In"=w327, "InArray"=w326, ".NET (Reference)"=w325) -> ("Error Out"=w330:errorcluster, "Image"=→"Image second camera":picture)  [unwired: 7 in]
          }
        }
      }
      frame "Init camera" {
        w355 = 1 items=["IS_DONT_WAIT", "IS_WAIT"] ("Wait")
        w382 = 0 items=["RGB 32"=0, "RGB 24"=1, "Y8 Monochrom"=6] ("Mode")
        # "SubVI Example for \nGetDefault Timing"
        # "SubVI Example for \nMemory allocation"
        # "SubVI Example for \nTiming"
        # "SubVI Example for \nCamera Init"
        # "Pixelformat"
        n214 = control-ref of="Init Camera 2"() -> (w350:refnum<vi>)
        n215 = control-ref of="Exit Camera 2"() -> (w348:refnum<vi>)
        n216 = property class="Bool"(reference=w350, "Disabled"=u8 2 ("Deaktiviert")) -> ()  [unwired: 1 in, 2 out]
        n217 = property class="Bool"(reference=w348, "Disabled"=u8 0 ("Deaktiviert")) -> ()  [unwired: 1 in, 2 out]
        n218 = call <instrlib>:"SubVI_Example_CameraInit.vi"("Error In"=w374, "Camera ID"="Camera ID 3", "Init Camera Flag"=TRUE, ".NET (Reference)"=w375) -> ("Error Out"=w379:errorcluster, ".NET (Reference)"=w353:refnum<k24>)  [unwired: 6 in]
        n219 = property class="Camera"(reference=w353, error in=w379) -> (error out=w380:errorcluster, "PixelFormat"=w381:refnum<k24>)  [unwired: 1 out]
        n220 = invoke class="PixelFormat" method="Set"(reference=w381, error in=w380, "mode"=w382) -> (reference out=w377:refnum<k24>, error out=w371:errorcluster, "Set"=w376:i32)  [unwired: 1 in, 1 out]
        n221 = invoke class="PixelFormat" method="ToString"(reference=w377, error in=w371) -> (error out=w370:errorcluster, "ToString"=w378:string)  [unwired: 1 in, 1 out]
        n222 = call <instrlib>:"Error_Handling.vi"("Error Code"=w376, "Error String"=w378, "Error In"=w370) -> ("Error Out"=w367:errorcluster)  [unwired: 8 in]
        n223 = call <instrlib>:"SubVI_Example_GetDefault_Timing.vi"(".NET (Reference)"=w353, "Error In"=w367) -> ("Pixelclock"=w364:i32, "Exposure time"=w365:dbl, "Framerate"=w366:dbl, "Error Out"=w363:errorcluster)  [unwired: 10 in]
        n224 = call <instrlib>:"SubVI_Example_Timing.vi"(".NET (Reference)"=w353, "Pixelclock"=w364, "Exposure time"=w365, "Framerate"=w366, "Error In"=w363) -> ("Error Out"=w369:errorcluster)  [unwired: 7 in, 3 out]
        n225 = call <instrlib>:"SubVI_Example_MemoryAllocation.vi"(".NET (Reference)"=w353, "Error In"=w369) -> ("Serial Number"=→"Serial Number 2":string, "Error Out"=w352:errorcluster)  [unwired: 13 in, 3 out]
        n226 = property class="Camera"(reference=w353, error in=w352) -> (error out=w361:errorcluster, "Acquisition"=w362:refnum<k24>)  [unwired: 1 out]
        n227 = invoke class="Acquisition" method="Capture"(reference=w362, error in=w361, "param"=w355) -> (reference out=w357:refnum<k24>, error out=w358:errorcluster, "Capture"=w356:i32)  [unwired: 1 in, 1 out]
        n228 = invoke class="Acquisition" method="ToString"(reference=w357, error in=w358) -> (error out=w360:errorcluster, "ToString"=w359:string)  [unwired: 1 in, 1 out]
        n229 = call <instrlib>:"Error_Handling.vi"("Error Code"=w356, "Error String"=w359, "Error In"=w360) -> ("Error Out"=w354:errorcluster)  [unwired: 8 in]
      }
    }
    n230 = case shown="Default" w150 {
      tunnel: w141 -> [w393 w424 w489]
      tunnel: w140 -> [w394 w423 w488]
      tunnel: [w403 w426 w468] -> w143
      tunnel: [w404 w425 w469] -> w147
      tunnel: [TRUE FALSE FALSE] -> w145
      frame "Exit camera" {
        # "Close .Net Referenz"
        # "Is acquisition running?"
        # "Stop Acquisition"
        # "Close Camera"
        n231 = control-ref of="Init Camera"() -> (w388:refnum<vi>)
        n232 = control-ref of="Exit Camera"() -> (w387:refnum<vi>)
        n233 = property class="Camera"(reference=w393, error in=w394) -> (error out=w402:errorcluster, "Acquisition"=w401:refnum<k24>)  [unwired: 1 out]
        n234 = property class="Bool"(reference=w388, "Disabled"=u8 0 ("Deaktiviert")) -> ()  [unwired: 1 in, 2 out]
        n235 = property class="Bool"(reference=w387, "Disabled"=u8 2 ("Deaktiviert")) -> ()  [unwired: 1 in, 2 out]
        n236 = invoke class="Acquisition" method="HasStarted"(reference=w401, error in=w402) -> (reference out=w395:refnum<k24>, error out=w398:errorcluster, "bValue"=w400:bool)  [unwired: 2 in, 1 out]
        n237 = invoke class="Acquisition" method="ToString"(reference=w395, error in=w398) -> (error out=w397:errorcluster, "ToString"=w396:string)  [unwired: 1 in, 1 out]
        n238 = call <instrlib>:"Error_Handling.vi"("Error String"=w396, "Error In"=w397) -> ("Error Out"=w399:errorcluster)  [unwired: 9 in]
        n239 = case shown="True" w400 {
          tunnel: [w412 w421] -> w391
          tunnel: w399 -> [w412 w422]
          tunnel: w393 -> [w411 w413]
          tunnel: [w411 w413] -> w392
          frame False {
          }
          frame True {
            n240 = property class="Camera"(reference=w413, error in=w422) -> (error out=w417:errorcluster, "Acquisition"=w418:refnum<k24>)  [unwired: 1 out]
            n241 = invoke class="Acquisition" method="Stop"(reference=w418, error in=w417) -> (reference out=w415:refnum<k24>, error out=w416:errorcluster, "Stop"=w414:i32)  [unwired: 1 in]
            n242 = invoke class="Acquisition" method="ToString"(reference=w415, error in=w416) -> (error out=w420:errorcluster, "ToString"=w419:string)  [unwired: 1 in, 1 out]
            n243 = call <instrlib>:"Error_Handling.vi"("Error Code"=w414, "Error String"=w419, "Error In"=w420) -> ("Error Out"=w421:errorcluster)  [unwired: 8 in]
          }
        }
        n244 = invoke class="Camera" method="Exit"(reference=w392, error in=w391) -> (reference out=w403:refnum<k24>, error out=w407:errorcluster, "Exit"=w406:i32)  [unwired: 1 in]
        n245 = invoke class="Camera" method="ToString"(reference=w403, error in=w407) -> (error out=w408:errorcluster, "ToString"=w409:string)  [unwired: 1 in, 1 out]
        n246 = call <instrlib>:"Error_Handling.vi"("Error Code"=w406, "Error String"=w409, "Error In"=w408) -> ("Error Out"=w405:errorcluster)  [unwired: 8 in]
        n247 = Close Reference ("Close Referenz")(reference=w403, error in (no error)=w405) -> (error out=w404:errorcluster)
      }
      frame Default {
        # "Has acquisition started?"
        n248 = property class="Camera"(reference=w424, error in=w423) -> (error out=w435:errorcluster, "Acquisition"=w434:refnum<k24>)  [unwired: 1 out]
        n249 = invoke class="Acquisition" method="HasStarted"(reference=w434, error in=w435) -> (reference out=w430:refnum<k24>, error out=w429:errorcluster, "HasStarted"=w428:i32, "bValue"=w433:bool)  [unwired: 2 in]
        n250 = invoke class="Acquisition" method="ToString"(reference=w430, error in=w429) -> (error out=w432:errorcluster, "ToString"=w431:string)  [unwired: 1 in, 1 out]
        n251 = call <instrlib>:"Error_Handling.vi"("Error Code"=w428, "Error String"=w431, "Error In"=w432) -> ("Error Out"=w427:errorcluster)  [unwired: 8 in]
        n252 = case shown="True" w433 {
          tunnel: [w438 w444] -> w425
          tunnel: w427 -> [w438 w443]
          tunnel: w424 -> [w437 w441]
          tunnel: [w437 w441] -> w426
          frame False {
            # "Show Image"
          }
          frame True {
            # "Memory"
            n253 = property class="Camera"(reference=w441, error in=w443) -> (error out=w446:errorcluster, "Memory"=w447:refnum<k24>)  [unwired: 1 out]
            n254 = invoke class="Memory" method="GetActive"(reference=w447, error in=w446) -> (reference out=w453:refnum<k24>, error out=w452:errorcluster, "GetActive"=w454:i32, "s32MemId"=w445:i32)  [unwired: 2 in]
            n255 = invoke class="Memory" method="ToString"(reference=w453, error in=w452) -> (error out=w450:errorcluster, "ToString"=w451:string)  [unwired: 1 in, 1 out]
            n256 = call <instrlib>:"Error_Handling.vi"("Error Code"=w454, "Error String"=w451, "Error In"=w450) -> ("Error Out"=w455:errorcluster)  [unwired: 8 in]
            n257 = property class="Camera"(reference=w441, error in=w455) -> (error out=w449:errorcluster, "Memory"=w448:refnum<k24>)  [unwired: 1 out]
            n258 = invoke class="Memory" method="CopyToArray"(reference=w448, error in=w449, "s32MemId"=w445) -> (reference out=w458:refnum<k24>, error out=w459:errorcluster, "CopyToArray"=w460:i32, "u8Image"=w440:u8[])  [unwired: 2 in, 1 out]
            n259 = invoke class="Memory" method="ToString"(reference=w458, error in=w459) -> (error out=w456:errorcluster, "ToString"=w457:string)  [unwired: 1 in, 1 out]
            n260 = call <instrlib>:"Error_Handling.vi"("Error Code"=w460, "Error String"=w457, "Error In"=w456) -> ("Error Out"=w442:errorcluster)  [unwired: 8 in]
            n261 = call <instrlib>:"ArrayToImage.vi"("Error In"=w442, "InArray"=w440, ".NET (Reference)"=w441) -> ("Error Out"=w444:errorcluster, "Image"=→"Image first camera":picture)  [unwired: 7 in]
          }
        }
      }
      frame "Init camera" {
        w470 = 1 items=["IS_DONT_WAIT", "IS_WAIT"] ("Wait")
        w496 = 0 items=["RGB 32"=0, "RGB 24"=1, "Y8 Monochrom"=6] ("Mode")
        # "SubVI Example for \nGetDefault Timing"
        # "SubVI Example for \nMemory allocation"
        # "SubVI Example for \nTiming"
        # "SubVI Example for \nCamera Init"
        # "Pixelformat"
        n262 = control-ref of="Init Camera"() -> (w464:refnum<vi>)
        n263 = control-ref of="Exit Camera"() -> (w462:refnum<vi>)
        n264 = call <instrlib>:"SubVI_Example_CameraInit.vi"("Error In"=w488, "Camera ID"="Camera ID 1", "Init Camera Flag"=TRUE, ".NET (Reference)"=w489) -> ("Error Out"=w493:errorcluster, ".NET (Reference)"=w468:refnum<k24>)  [unwired: 6 in]
        n265 = property class="Bool"(reference=w464, "Disabled"=u8 2 ("Deaktiviert")) -> ()  [unwired: 1 in, 2 out]
        n266 = property class="Bool"(reference=w462, "Disabled"=u8 0 ("Deaktiviert")) -> ()  [unwired: 1 in, 2 out]
        n267 = property class="Camera"(reference=w468, error in=w493) -> (error out=w494:errorcluster, "PixelFormat"=w495:refnum<k24>)  [unwired: 1 out]
        n268 = invoke class="PixelFormat" method="Set"(reference=w495, error in=w494, "mode"=w496) -> (reference out=w491:refnum<k24>, error out=w485:errorcluster, "Set"=w490:i32)  [unwired: 1 in, 1 out]
        n269 = invoke class="PixelFormat" method="ToString"(reference=w491, error in=w485) -> (error out=w484:errorcluster, "ToString"=w492:string)  [unwired: 1 in, 1 out]
        n270 = call <instrlib>:"Error_Handling.vi"("Error Code"=w490, "Error String"=w492, "Error In"=w484) -> ("Error Out"=w481:errorcluster)  [unwired: 8 in]
        n271 = call <instrlib>:"SubVI_Example_GetDefault_Timing.vi"(".NET (Reference)"=w468, "Error In"=w481) -> ("Pixelclock"=w478:i32, "Exposure time"=w479:dbl, "Framerate"=w480:dbl, "Error Out"=w466:errorcluster)  [unwired: 10 in]
        n272 = call <instrlib>:"SubVI_Example_Timing.vi"(".NET (Reference)"=w468, "Pixelclock"=w478, "Exposure time"=w479, "Framerate"=w480, "Error In"=w466) -> ("Error Out"=w483:errorcluster)  [unwired: 7 in, 3 out]
        n273 = call <instrlib>:"SubVI_Example_MemoryAllocation.vi"(".NET (Reference)"=w468, "Error In"=w483) -> ("Serial Number"=→"Serial Number 1":string, "Error Out"=w467:errorcluster)  [unwired: 13 in, 3 out]
        n274 = property class="Camera"(reference=w468, error in=w467) -> (error out=w476:errorcluster, "Acquisition"=w477:refnum<k24>)  [unwired: 1 out]
        n275 = invoke class="Acquisition" method="Capture"(reference=w477, error in=w476, "param"=w470) -> (reference out=w472:refnum<k24>, error out=w473:errorcluster, "Capture"=w471:i32)  [unwired: 1 in, 1 out]
        n276 = invoke class="Acquisition" method="ToString"(reference=w472, error in=w473) -> (error out=w475:errorcluster, "ToString"=w474:string)  [unwired: 1 in, 1 out]
        n277 = call <instrlib>:"Error_Handling.vi"("Error Code"=w471, "Error String"=w474, "Error In"=w475) -> ("Error Out"=w469:errorcluster)  [unwired: 8 in]
      }
    }
    n278 = case shown="False" "steps /\n continuous \ntoggle" {
      tunnel: w114 -> [w171 w247]
      tunnel: w113 -> [w170 w246]
      tunnel: [w189 w253] -> w112
      tunnel: [w162 w259] -> w102
      tunnel: "up a1" -> [w188 w255]
      tunnel: "down a1" -> [w186 w254]
      tunnel: "up all" -> [w169 w242]
      tunnel: "down all" -> [w168 w243]
      tunnel: "down a3" -> [w176 w251]
      tunnel: "up a3" -> [w177 w250]
      tunnel: "down a2" -> [w174 w245]
      tunnel: "up a2" -> [w175 w244]
      tunnel: w107 -> [_ w257]
      tunnel: [_ w258] -> w111
      tunnel: [_ w238] -> w110
      tunnel: w106 -> [_ w235]
      tunnel: [_ w236] -> w108
      tunnel: w104 -> [_ w233]
      tunnel: [_ w237] -> w109
      tunnel: w105 -> [_ w234]
      frame False {
        n279 = flat-sequence {
          tunnel: w171 -> [w204]
          tunnel: w170 -> [w207]
          tunnel: w177 -> [w202]
          tunnel: "a3" ("Combo Box") -> [w200]
          tunnel: "Step size" -> [w203]
          tunnel: w176 -> [w201]
          tunnel: [w206] -> w180
          tunnel: [w205] -> w179
          tunnel: [w209] -> _
          tunnel: [w210] -> w164
          tunnel: w180 -> [w210]
          tunnel: w179 -> [w209]
          frame #0 {
            n280 = call "Picomotor step single.vi"("Step size"=w203, "Combo Box"=w200, "error in (no error)"=w207, "down a1"=w201, "up a1"=w202, "VISA Refnum in"=w204) -> ("error out"=w206:errorcluster, "VISA Refnum out"=w205:refnum<visa-resource-name>)  [unwired: 4 in]
          }
          frame #1 {
            n281 = Wait (ms)(milliseconds to wait=u32 100) -> ()  [unwired: 1 out]
          }
        }
        n282 = flat-sequence {
          tunnel: w171 -> [w226]
          tunnel: w170 -> [w229]
          tunnel: w188 -> [w224]
          tunnel: "a1" ("Combo Box") -> [w222]
          tunnel: "Step size" -> [w225]
          tunnel: w186 -> [w223]
          tunnel: [w228] -> w185
          tunnel: [w227] -> w184
          tunnel: [w231] -> w189
          tunnel: [w232] -> w166
          tunnel: w185 -> [w232]
          tunnel: w184 -> [w231]
          frame #0 {
            n283 = call "Picomotor step single.vi"("Step size"=w225, "Combo Box"=w222, "error in (no error)"=w229, "down a1"=w223, "up a1"=w224, "VISA Refnum in"=w226) -> ("error out"=w228:errorcluster, "VISA Refnum out"=w227:refnum<visa-resource-name>)  [unwired: 4 in]
          }
          frame #1 {
            n284 = Wait (ms)(milliseconds to wait=u32 100) -> ()  [unwired: 1 out]
          }
        }
        n285 = flat-sequence {
          tunnel: w171 -> [w215]
          tunnel: w170 -> [w218]
          tunnel: w175 -> [w213]
          tunnel: "a2" ("Combo Box") -> [w211]
          tunnel: "Step size" -> [w214]
          tunnel: w174 -> [w212]
          tunnel: [w217] -> w183
          tunnel: [w216] -> w182
          tunnel: [w220] -> _
          tunnel: [w221] -> w165
          tunnel: w183 -> [w221]
          tunnel: w182 -> [w220]
          frame #0 {
            n286 = call "Picomotor step single.vi"("Step size"=w214, "Combo Box"=w211, "error in (no error)"=w218, "down a1"=w212, "up a1"=w213, "VISA Refnum in"=w215) -> ("error out"=w217:errorcluster, "VISA Refnum out"=w216:refnum<visa-resource-name>)  [unwired: 4 in]
          }
          frame #1 {
            n287 = Wait (ms)(milliseconds to wait=u32 100) -> ()  [unwired: 1 out]
          }
        }
        n288 = flat-sequence {
          tunnel: [w196] -> w173
          tunnel: [w195] -> w172
          tunnel: w171 -> [w194]
          tunnel: w170 -> [w193]
          tunnel: w169 -> [w192]
          tunnel: w168 -> [w191]
          tunnel: "Step size" -> [w190]
          tunnel: [w198] -> _
          tunnel: [w199] -> w163
          tunnel: w173 -> [w199]
          tunnel: w172 -> [w198]
          frame #0 {
            n289 = call "Picomotor step multi.vi"("Step size"=w190, "error in (no error)"=w193, "down a1"=w191, "up a1"=w192, "VISA Refnum in"=w194) -> ("error out"=w196:errorcluster, "VISA Refnum out"=w195:refnum<visa-resource-name>)  [unwired: 5 in]
          }
          frame #1 {
            n290 = Wait (ms)(milliseconds to wait=u32 100) -> ()  [unwired: 1 out]
          }
        }
        n291 = Merge Errors(w166, w165, w164, w163) -> (w162:errorcluster)
      }
      frame True {
        n292 = call "Picomotor single motor continuous.vi"("Enum"=w257, "Combo Box"="a1", "error in (no error)"=w246, "down"=w254, "up"=w255, "VISA Refnum in"=w247) -> ("error out"=w252:errorcluster, "Numeric"=w258:i32, "VISA Refnum out"=w253:refnum<visa-resource-name>)  [unwired: 3 in]
        n293 = call "Picomotor single motor continuous.vi"("Enum"=w234, "Combo Box"="a3", "error in (no error)"=w246, "down"=w251, "up"=w250, "VISA Refnum in"=w247) -> ("error out"=w240:errorcluster, "Numeric"=w237:i32)  [unwired: 3 in, 1 out]
        n294 = call "Picomotor single motor continuous.vi"("Enum"=w235, "Combo Box"="a2", "error in (no error)"=w246, "down"=w245, "up"=w244, "VISA Refnum in"=w247) -> ("error out"=w241:errorcluster, "Numeric"=w238:i32)  [unwired: 3 in, 1 out]
        n295 = call "Picomotor all motors continuous.vi"("Enum"=w233, "error in (no error)"=w246, "down"=w243, "up"=w242, "VISA Refnum in"=w247) -> ("error out"=w239:errorcluster, "Numeric"=w236:i32)  [unwired: 4 in, 1 out]
        n296 = Merge Errors(w252, w241, w240, w239) -> (w259:errorcluster)
      }
    }
    n297 = call <instrlib>:"SubVI_Example_SyncEventLoop.vi"("Error In"=w134, "use sync"=w132, ".NET (Reference)"=w130) -> ("Error Out"=w129:errorcluster, "Synchronize (ms)"=w133:dbl)  [unwired: 7 in]
    "Error Camera 2" <- w129
    n298 = call <instrlib>:"SubVI_Example_SyncEventLoop.vi"("Error In"=w147, "use sync"=w145, ".NET (Reference)"=w143) -> ("Error Out"=w142:errorcluster, "Synchronize (ms)"=w146:dbl)  [unwired: 7 in]
    "Error Camera 1" <- w142
    n299 = Wait Until Next ms Multiple(millisecond multiple=w146) -> ()  [unwired: 1 out]
    n300 = Wait Until Next ms Multiple(millisecond multiple=w133) -> ()  [unwired: 1 out]
    n301 = case shown="False" "stop" {
      tunnel: w112 -> [w262 w267]
      tunnel: w102 -> [w261 w266]
      tunnel: [w262 w265] -> w101
      tunnel: [w261 w264] -> w103
      tunnel: [w260 w263] -> w125
      tunnel: "stop" -> [w260 w263]
      frame False {
      }
      frame True {
        n302 = call "Picomotor Write.vi"("error in (no error)"=w266, "String 3"="sto", "VISA Refnum in"=w267) -> ("error out"=w264:errorcluster, "VISA Refnum out"=w265:refnum<visa-resource-name>)  [unwired: 6 in, 1 out]
      }
    }
    n303 = Merge Errors(w103, w102) -> (w126:errorcluster)
  }
  n304 = VISA Close(VISA resource name=w1, error in (no error)=w2) -> (error out=→"error":errorcluster)
